vi "signal_analysis.vi"() -> ()   [LabVIEW 2020]
uses:
  <vilib>/express/express analysis/Spectral/Block/exnSpectralBlock spectral measurements PSD poly.vi
  <vilib>/express/express analysis/Spectral/Block/exnSpectralBlock spectral measurements PSD WFM.vi
  <vilib>/express/express analysis/Spectral/XNode/ExpressSpectralMeasurementsBlockNode.xnode
  <vilib>/measure/NI_MABase.lvlib
panel:
  out "Filtered Signal":dynamicdata(graph)
  out "PSD Spectral Display":cluster{"f0":dbl, "df":dbl, "magnitude":dbl[]}(graph)
  out "Multitude":waveform(dbl)(graph)
  out "Sine 2 & Sine 3":waveform(dbl)(graph)
  out "Sine 1 & Sine 2":waveform(dbl)(graph)
  out "Sine 1":waveform(dbl)(graph)
  out "Sine 2":waveform(dbl)(graph)
  out "Sine 3":waveform(dbl)(graph)
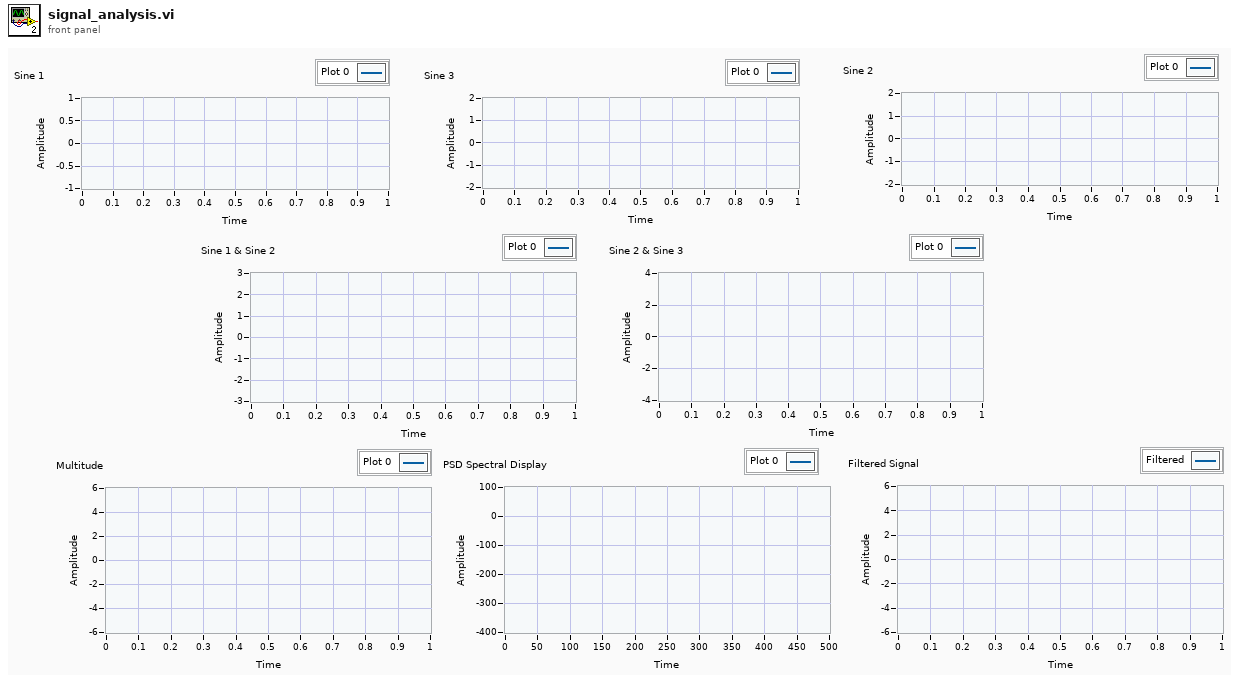
[diagram p1: front panel]
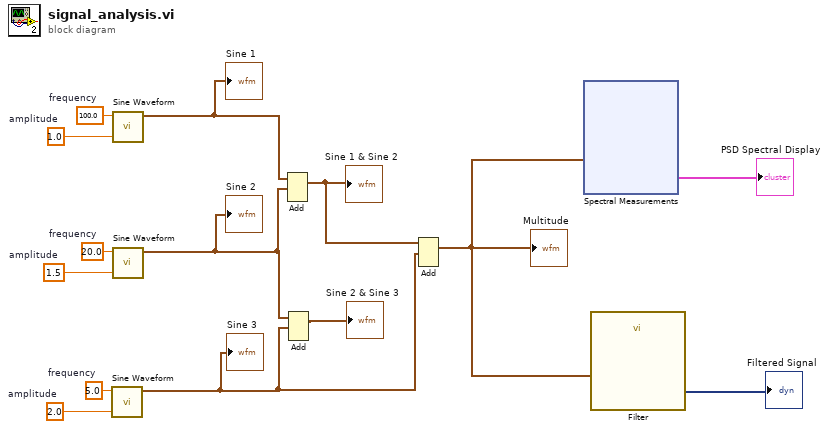
[diagram p0: block diagram]
diagram:
  w9 = 2.0  # amplitude
  w10 = 5.0  # frequency
  w11 = 1.5  # amplitude
  w12 = 20.0  # frequency
  w13 = 1.0  # amplitude
  w14 = 100.0  # frequency
  n1 = call <vilib>:"Sine Waveform.vi"("amplitude"=w9, "frequency"=w10) -> ("signal out"=w8:waveform(dbl))  [unwired: 8 in, 1 out]
  "Sine 3" <- w8
  n2 = call <vilib>:"Sine Waveform.vi"("amplitude"=w13, "frequency"=w14) -> ("signal out"=w6:waveform(dbl))  [unwired: 8 in, 1 out]
  "Sine 1" <- w6
  n3 = call <vilib>:"Sine Waveform.vi"("amplitude"=w11, "frequency"=w12) -> ("signal out"=w7:waveform(dbl))  [unwired: 8 in, 1 out]
  "Sine 2" <- w7
  n4 = Add(1:w7, 2:w6) -> (0:w5:waveform(dbl))  [unwired: 1 in, 1 out]
  "Sine 1 & Sine 2" <- w5
  n5 = Add(1:w8, 2:w7) -> (0:→"Sine 2 & Sine 3":waveform(dbl))  [unwired: 1 in, 1 out]
  n6 = Add(1:w8, 2:w5) -> (0:w3:waveform(dbl))  [unwired: 1 in, 1 out]
  "Multitude" <- w3
  n7 = xnode "Spectral Measurements"("Signals"=w3) -> ("PSD"=→"PSD Spectral Display":cluster{"f0":dbl, "df":dbl, "magnitude":dbl[]})  [unwired: 1 in, 1 out]
  n8 = call "Filter"("Signal"=w3) -> ("Filtered Signal"=→"Filtered Signal":dynamicdata)  [unwired: 9 in, 1 out]
